vi "SW_Get_save_paths.vi"(3 "error in (no error)":errorcluster, 4 "Final file name prefix":string="SavedTrack", 5 "Temporary file name prefix":string="TrackTemp") -> (0 "error out":errorcluster, 2 "Output cluster of paths":T1)   [LabVIEW 2016]
uses:
  <vilib>/Utility/sysdir.llb/System Directory Type.ctl
panel:
  out "Final output path":path
  out "Background picture output path":path
  out "Recording settings output path":path
  out "Temporary csv output path":path
  out "date/time string":string
  out "Temporary file output path":path
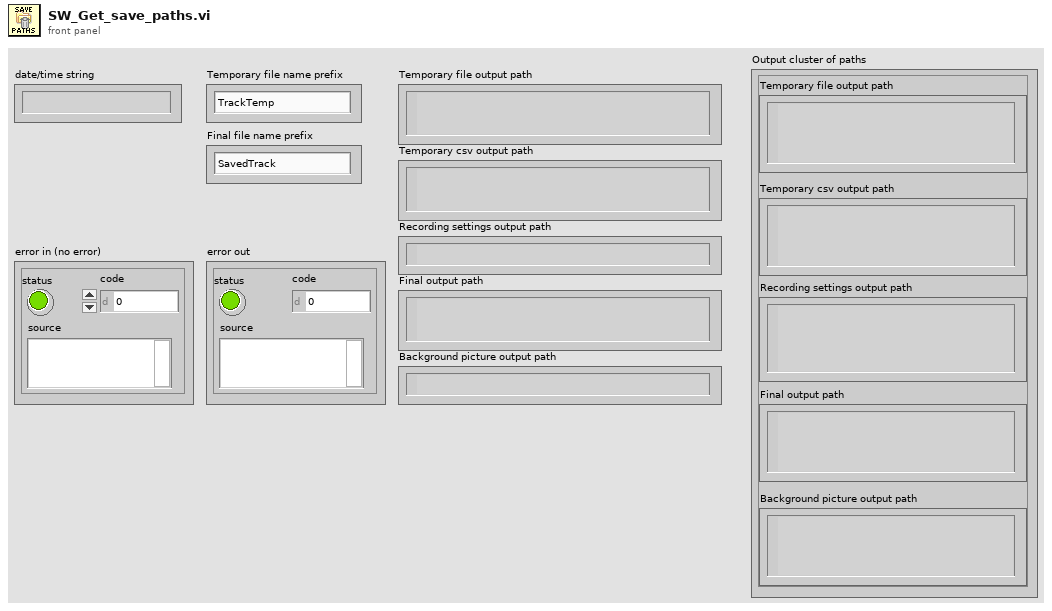
[diagram p1: front panel]
types:
  T1 = cluster{"Temporary file output path":path, "Temporary csv output path":path, "Recording settings output path":path, "Final output path":path, "Background picture output path":path}
  T2 = typedef "System Directory Type.ctl" = i32
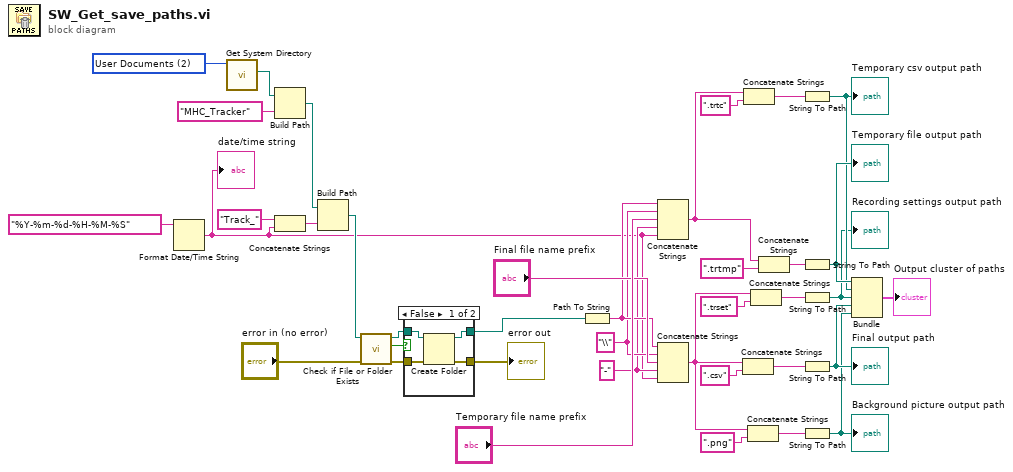
[diagram p0: block diagram]
diagram:
  w36 = T2 2 items=["User Home"=0, "User Desktop"=1, "User Documents"=2, "User Application Data"=3, "User Preferences"=4, "User Temporary"=5, "Public Documents"=6, "Public Application Data"=7, "Public Preferences"=8, "Public Cache"=13, "System Core Libraries"=9, "System Installed Libraries"=10, "Application Files"=11, "Boot Volume Root"=12] ("system directory type")
  w21 = "-" ("string")
  w22 = "\\" ("string")
  n1 = Format Date/Time String(time format string (%c)="%Y-%m-%d-%H-%M-%S") -> (date/time string=w2:string)  [unwired: 2 in]
  "date/time string" <- w2
  n2 = call <vilib>:"Get System Directory.vi"("system directory type"=w36) -> ("system directory"=w34:path)  [unwired: 10 in]
  n3 = Build Path(base path=w34, name or relative path="MHC_Tracker" ("string")) -> (appended path=w6:path)
  n4 = Concatenate Strings("Track_" ("string"), w2) -> (w3:string)
  n5 = Build Path(base path=w6, name or relative path=w3) -> (appended path=w5:path)
  n6 = call <vilib>:"Check if File or Folder Exists.vi"("error in (no error)"="error in (no error)", "path"=w5) -> ("error out"=w31:errorcluster, "file or folder exists?"=w33:bool, "dup path"=w32:path)  [unwired: 7 in]
  n7 = case shown="False" w33 {
    tunnel: w32 -> [w41 w44]
    tunnel: w31 -> [w42 w43]
    tunnel: [w39 w44] -> w8
    tunnel: [w40 w43] -> w7
    frame False {
      n8 = Create Folder(path (use dialog)=w41, error in=w42) -> (created path=w39:path, error out=w40:errorcluster)  [unwired: 1 in, 1 out]
    }
    frame True {
    }
  }
  "error out" <- w7
  n9 = Path To String(path=w8) -> (string=w23:string)
  n10 = Concatenate Strings(w23, w22, "Temporary file name prefix", w21, w2) -> (w12:string)
  n11 = Concatenate Strings(w23, w22, "Final file name prefix", w21, w2) -> (w9:string)
  n12 = Concatenate Strings(w9, ".csv" ("string")) -> (w26:string)
  n13 = Concatenate Strings(w12, ".trtc" ("string")) -> (w27:string)
  n14 = Concatenate Strings(w9, ".png" ("string")) -> (w13:string)
  n15 = Concatenate Strings(w9, ".trset" ("string")) -> (w11:string)
  n16 = Concatenate Strings(w12, ".trtmp" ("string")) -> (w29:string)
  n17 = String To Path(string=w27) -> (path=w19:path)
  "Temporary csv output path" <- w19
  n18 = String To Path(string=w29) -> (path=w20:path)
  "Temporary file output path" <- w20
  n19 = String To Path(string=w11) -> (path=w18:path)
  "Recording settings output path" <- w18
  n20 = String To Path(string=w26) -> (path=w17:path)
  "Final output path" <- w17
  n21 = String To Path(string=w13) -> (path=w16:path)
  "Background picture output path" <- w16
  n22 = Bundle(w20, w19, w18, w17, w16) -> (→"Output cluster of paths":cluster{path, path, path, path, path})  [unwired: 1 in]
